vi "Check If Pixels Belong In Sector.vi"() -> (3 "FIFO Timeout?":bool)   [LabVIEW 2013]
uses:
  Globals/Pixel Location Global.vi
  Globals/Accumulated Sector Intensity.vi
  <vilib>/rvi/FIFO/Fifo_Resource/nirvififoEmulationGetNumberOfElementsToWriteFpgaImpl.vi
  <vilib>/rvi/DataTransferAndStorage/Container/Common/niFpgaContainerGetUniqueNameForEmu.vi
  <vilib>/rvi/FIFO/Fifo_Resource/nirvififoEmulationGetNumberOfElementsToReadFpgaImpl.vi
  Globals/Sector Parameter Global.vi
  <vilib>/rvi/FIFO/Fifo_Resource/nirvififoEmulationReadFpgaImpl.vi
  <vilib>/rvi/FIFO/Fifo_Resource/nirvififoEmulationWriteFpgaImpl.vi
  <vilib>/rvi/DataTransferAndStorage/Container/XNode/niFpgaContainer.xnode
  <vilib>/rvi/FIFO/Fifo_Resource/nirvififoEmulationGetNumberOfElementsToWrite.vi
  <vilib>/rvi/FIFO/Fifo_Resource/nirvififoEmulationGetNumberOfElementsToRead.vi
  <vilib>/rvi/FIFO/Fifo_Resource/nirvififoEmulationRead.vi
  <vilib>/rvi/FIFO/Fifo_Resource/nirvififoEmulationWrite.vi
panel:
  out "Number of Elements to Write 4":u32
  out "Number of Elements to Write 3":u32
  out "Number of Elements to Write 2":u32
  out "Number of Elements to Write":u32
  out "Number of Elements to Read 4":u32
  out "Number of Elements to Read 3":u32
  out "Number of Elements to Read 2":u32
  out "Number of Elements to Read":u32
  out "End of  Data?":bool
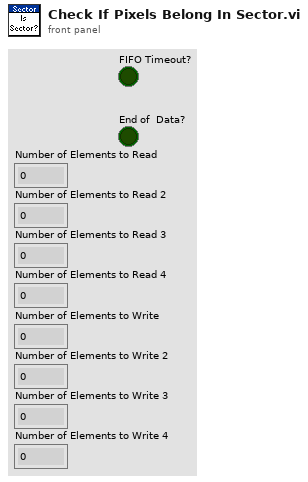
[diagram p1: front panel]
types:
  T1 = cluster{"Pixel Value":u8, "X":fxp<+,11,11>, "Y":fxp<+,11,11>}
  T2 = typedef "Sector Parameter Cluster.ctl" = cluster{"Start Angle":fxp<+/-,17,2>, "End Angle":fxp<+/-,17,2>, "Inner Radius":u16, "Outter Radius":u16, "Hinge X":u16, "Hinge Y":u16, "NumWingSectors":u8}
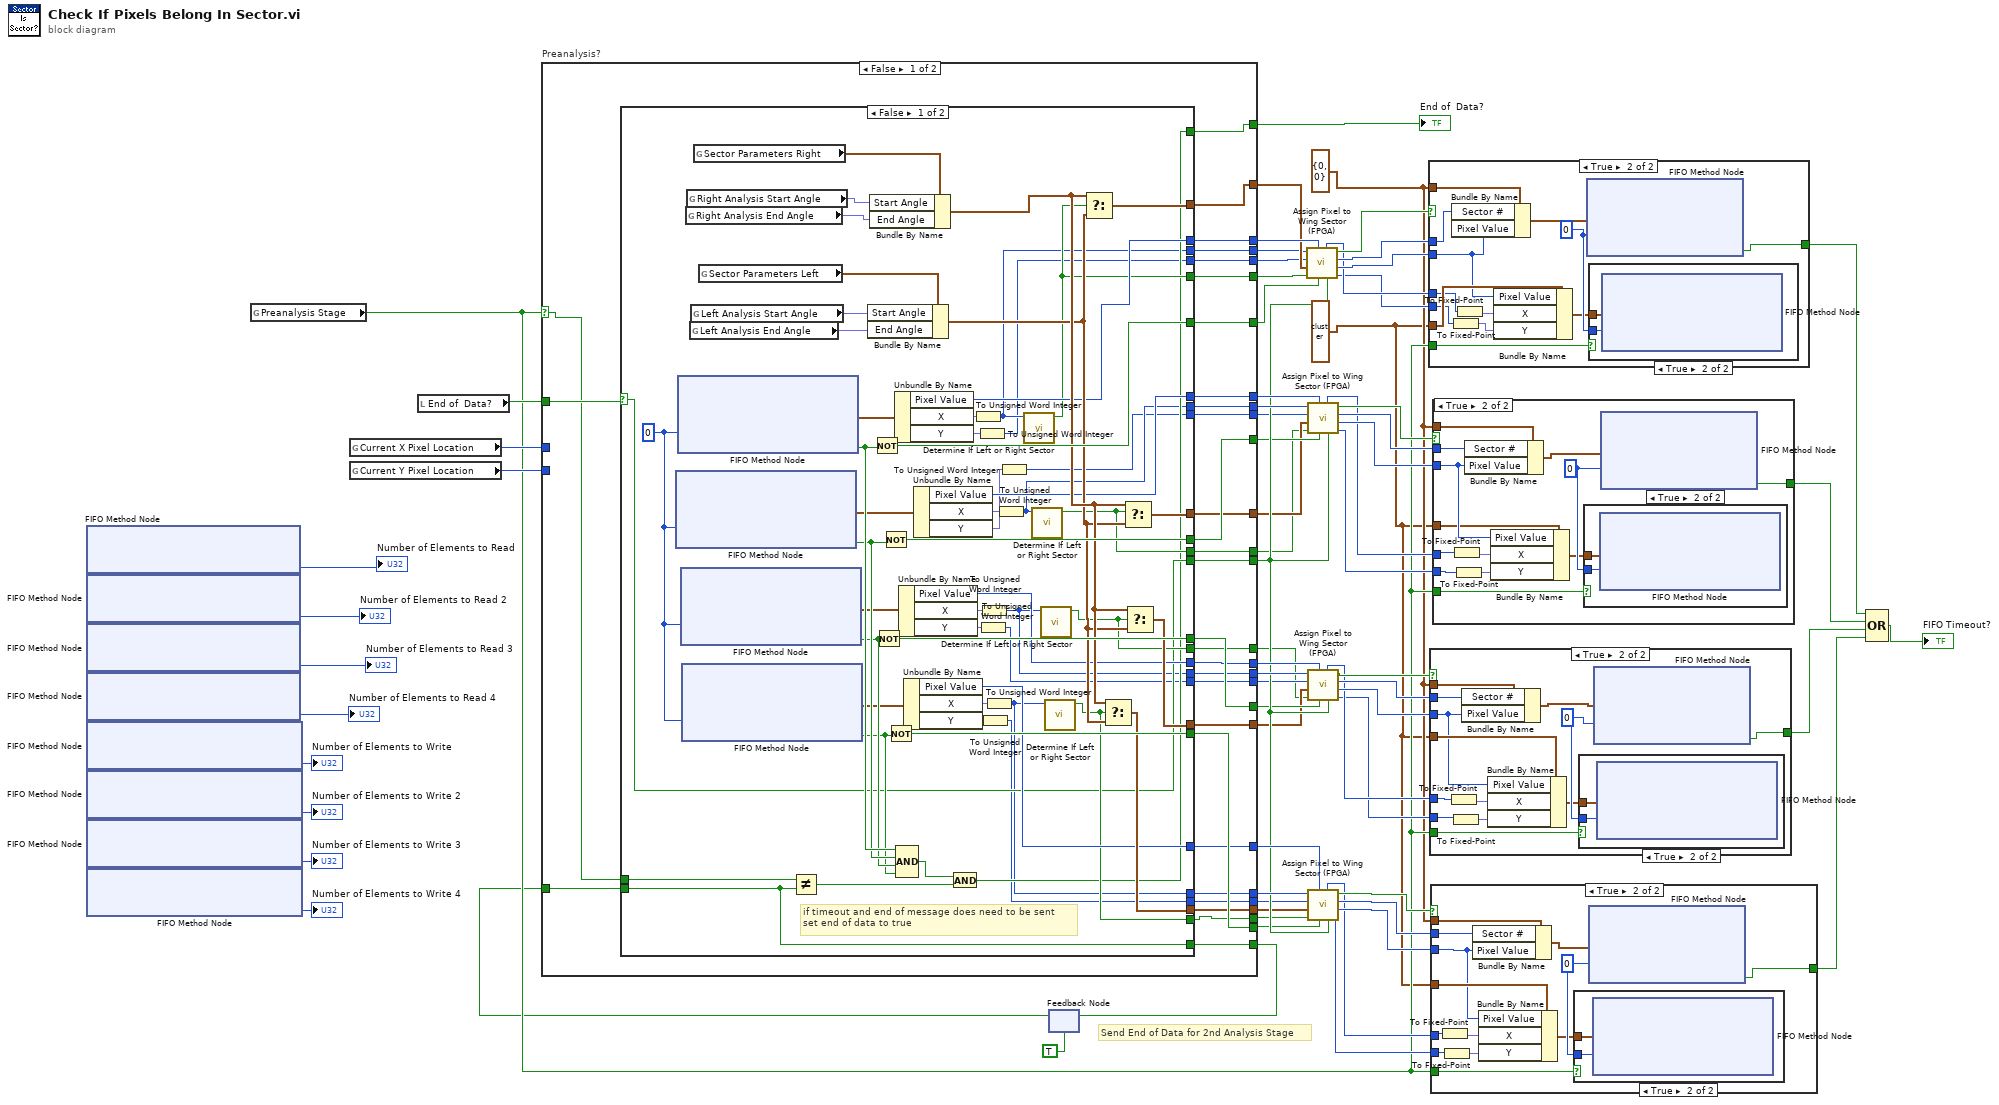
[diagram p0: block diagram]
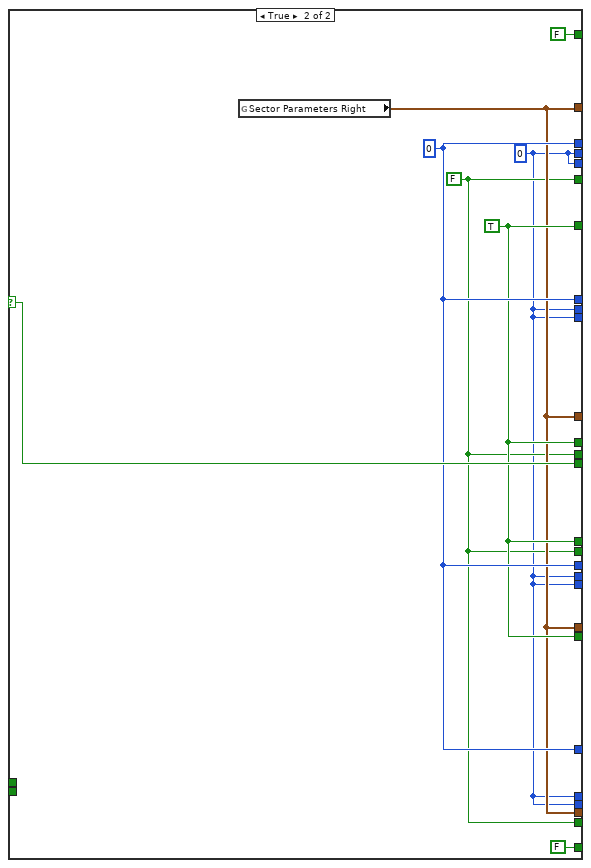
[diagram p2: hidden frame]
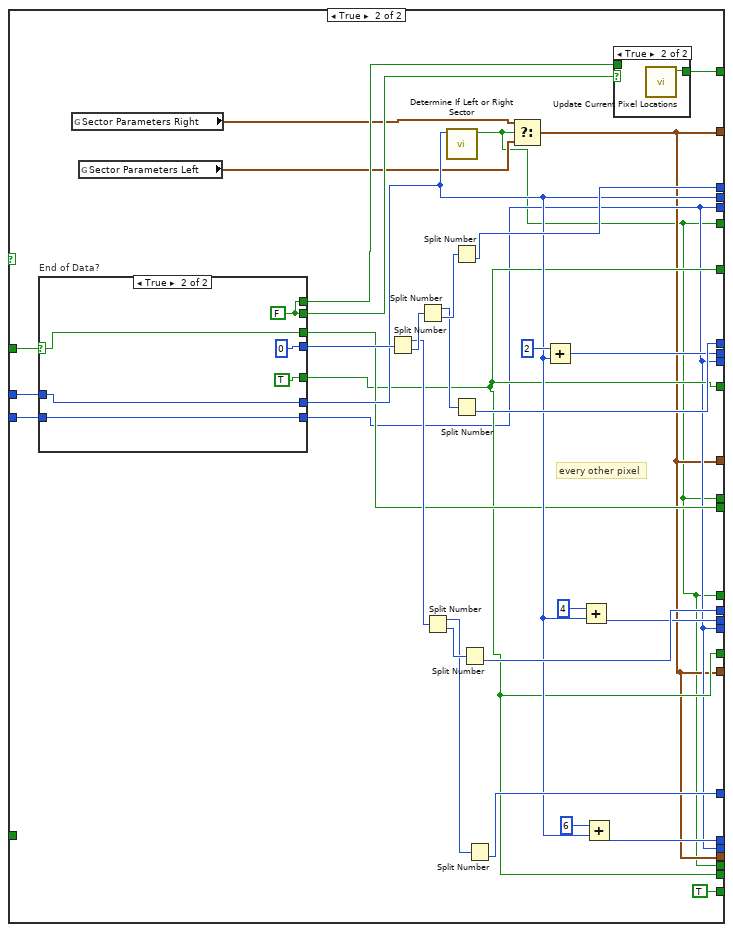
[diagram p3: hidden frame]
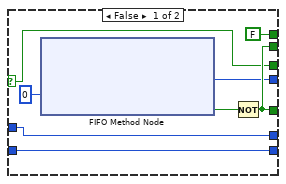
[diagram p4: hidden frame]
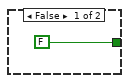
[diagram p6: hidden frame]
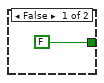
[diagram p8: hidden frame]
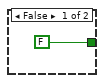
[diagram p10: hidden frame]
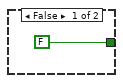
[diagram p12: hidden frame]
diagram:
  w9 = T1 {"Pixel Value"=0, "X"=0.0, "Y"=0.0} ("Element")
  w10 = cluster{"Sector #":u8, "Pixel Value":u8} {"Sector #"=0, "Pixel Value"=0} ("Element")
  # "Send End of Data for 2nd Analysis Stage"
  n1 = xnode ("FIFO Method Node")() -> ("Number of Elements to Read"=→"Number of Elements to Read":u32)  [unwired: 1 in, 1 out]
  n2 = xnode ("FIFO Method Node")() -> ("Number of Elements to Read"=→"Number of Elements to Read 2":u32)  [unwired: 1 in, 1 out]
  n3 = xnode ("FIFO Method Node")() -> ("Number of Elements to Read"=→"Number of Elements to Read 3":u32)  [unwired: 1 in, 1 out]
  n4 = xnode ("FIFO Method Node")() -> ("Number of Elements to Read"=→"Number of Elements to Read 4":u32)  [unwired: 1 in, 1 out]
  n5 = xnode ("FIFO Method Node")() -> ("Number of Elements to Write"=→"Number of Elements to Write":u32)  [unwired: 1 in, 1 out]
  n6 = xnode ("FIFO Method Node")() -> ("Number of Elements to Write"=→"Number of Elements to Write 2":u32)  [unwired: 1 in, 1 out]
  n7 = xnode ("FIFO Method Node")() -> ("Number of Elements to Write"=→"Number of Elements to Write 3":u32)  [unwired: 1 in, 1 out]
  n8 = xnode ("FIFO Method Node")() -> ("Number of Elements to Write"=→"Number of Elements to Write 4":u32)  [unwired: 1 in, 1 out]
  n9 = global read "Accumulated Sector Intensity.vi" "Preanalysis Stage"() -> (w26:bool)
  n10 = global read "Pixel Location Global.vi" "Current X Pixel Location"() -> (w37:u16)
  n11 = global read "Pixel Location Global.vi" "Current Y Pixel Location"() -> (w39:u16)
  n12 = local read "End of  Data?"() -> (w41:bool)
  n13 = feedback #1(TRUE) -> (w12:bool)
  n14 = case "Preanalysis?" shown="False" w26 {
    selector: w26 -> [w70 _]
    tunnel: [w93 w193] -> w68
    tunnel: [w75 w163] -> w50
    tunnel: [w87 w185] -> w49
    tunnel: [w86 w184] -> w48
    tunnel: [w85 w183] -> w47
    tunnel: [w84 w182] -> w46
    tunnel: [w82 w178] -> w45
    tunnel: [w81 w177] -> w44
    tunnel: [w80 w176] -> w43
    tunnel: [w91 w164] -> w42
    tunnel: [w97 w166] -> w27
    tunnel: w41 -> [w98 w173]
    tunnel: [w79 w165] -> w40
    tunnel: w39 -> [_ w172]
    tunnel: [w83 w171] -> w38
    tunnel: w37 -> [_ w170]
    tunnel: [w92 w169] -> w36
    tunnel: [w96 w166] -> w25
    tunnel: [w95 w166] -> w24
    tunnel: [w94 w166] -> w23
    tunnel: [w90 w164] -> w22
    tunnel: [w89 w164] -> w21
    tunnel: [w88 w164] -> w20
    tunnel: [w78 w165] -> w19
    tunnel: [w77 w165] -> w18
    tunnel: [w76 w165] -> w17
    tunnel: [w74 w163] -> w16
    tunnel: [w73 w163] -> w15
    tunnel: [w72 w163] -> w14
    tunnel: w12 -> [w71 _]
    tunnel: [w69 TRUE] -> w11
    frame False {
      n15 = case shown="False" w98 {
        selector: w98 -> [w116 w160]
        tunnel: [w146 w158] -> w97
        tunnel: [w145 w158] -> w96
        tunnel: [w144 w158] -> w95
        tunnel: [w143 w158] -> w94
        tunnel: [w112 FALSE] -> w93
        tunnel: [w116 w160] -> w92
        tunnel: [w138 w157] -> w91
        tunnel: [w137 w157] -> w90
        tunnel: [w136 w157] -> w89
        tunnel: [w133 w157] -> w88
        tunnel: [w132 w159] -> w87
        tunnel: [w131 w159] -> w86
        tunnel: [w130 w159] -> w85
        tunnel: [w129 w159] -> w84
        tunnel: [w110 w155] -> w83
        tunnel: [w108 w155] -> w82
        tunnel: [w106 w155] -> w81
        tunnel: [w104 w155] -> w80
        tunnel: [w109 w155] -> w79
        tunnel: [w107 w155] -> w78
        tunnel: [w105 w155] -> w77
        tunnel: [w103 w155] -> w76
        tunnel: [w120 w156] -> w75
        tunnel: [w119 w156] -> w74
        tunnel: [w118 w156] -> w73
        tunnel: [w117 w156] -> w72
        tunnel: w71 -> [w111 _]
        tunnel: w70 -> [w115 _]
        tunnel: [w111 FALSE] -> w69
        frame False {
          w147 = 0 ("Timeout")
          # "if timeout and end of message does need to be sent\nset end of data to true"
          n16 = xnode ("FIFO Method Node")("Timeout"=w147) -> ("Element"=w102:T1, "Timed Out?"=w141:bool)  [unwired: 1 in, 1 out]
          n17 = xnode ("FIFO Method Node")("Timeout"=w147) -> ("Element"=w101:T1, "Timed Out?"=w142:bool)  [unwired: 1 in, 1 out]
          n18 = xnode ("FIFO Method Node")("Timeout"=w147) -> ("Element"=w100:T1, "Timed Out?"=w140:bool)  [unwired: 1 in, 1 out]
          n19 = xnode ("FIFO Method Node")("Timeout"=w147) -> ("Element"=w99:T1, "Timed Out?"=w139:bool)  [unwired: 1 in, 1 out]
          n20 = global read "Sector Parameter Global.vi" "Right Analysis End Angle"() -> (w151:fxp<+/-,17,2>)
          n21 = global read "Sector Parameter Global.vi" "Right Analysis Start Angle"() -> (w152:fxp<+/-,17,2>)
          n22 = global read "Sector Parameter Global.vi" "Left Analysis End Angle"() -> (w148:fxp<+/-,17,2>)
          n23 = global read "Sector Parameter Global.vi" "Left Analysis Start Angle"() -> (w149:fxp<+/-,17,2>)
          n24 = global read "Sector Parameter Global.vi" "Sector Parameters Right"() -> (w153:T2)
          n25 = global read "Sector Parameter Global.vi" "Sector Parameters Left"() -> (w150:T2)
          n26 = Not Equal?(x=w115, y=w111) -> (x != y?=w113:bool)
          n27 = Bundle By Name(cluster=w150, "Start Angle"=w149, "End Angle"=w148) -> (w134:T2)
          n28 = Bundle By Name(cluster=w153, "Start Angle"=w152, "End Angle"=w151) -> (w135:T2)
          n29 = Not(x=w142) -> (.not. x?=w143:bool)
          n30 = Not(x=w140) -> (.not. x?=w145:bool)
          n31 = Not(x=w141) -> (.not. x?=w144:bool)
          n32 = Not(x=w139) -> (.not. x?=w146:bool)
          n33 = Unbundle By Name(w101) -> ("Pixel Value"=w132:u8, "X"=w128:fxp<+,11,11>, "Y"=w124:fxp<+,11,11>)
          n34 = Compound Arithmetic op=AND(w142, w141, w140, w139) -> (w114:bool)
          n35 = Unbundle By Name(w100) -> ("Pixel Value"=w130:u8, "X"=w126:fxp<+,11,11>, "Y"=w122:fxp<+,11,11>)
          n36 = Unbundle By Name(w99) -> ("Pixel Value"=w129:u8, "X"=w125:fxp<+,11,11>, "Y"=w121:fxp<+,11,11>)
          n37 = Unbundle By Name(w102) -> ("Pixel Value"=w131:u8, "X"=w127:fxp<+,11,11>, "Y"=w123:fxp<+,11,11>)
          n38 = And(x=w114, y=w113) -> (x .and. y?=w112:bool)
          n39 = To Unsigned Word Integer(number=w128) -> (unsigned 16bit integer=w110:u16)
          n40 = To Unsigned Word Integer(number=w124) -> (unsigned 16bit integer=w109:u16)
          n41 = To Unsigned Word Integer(number=w122) -> (unsigned 16bit integer=w105:u16)
          n42 = To Unsigned Word Integer(number=w126) -> (unsigned 16bit integer=w106:u16)
          n43 = To Unsigned Word Integer(number=w121) -> (unsigned 16bit integer=w103:u16)
          n44 = To Unsigned Word Integer(number=w125) -> (unsigned 16bit integer=w104:u16)
          n45 = To Unsigned Word Integer(number=w127) -> (unsigned 16bit integer=w108:u16)
          n46 = To Unsigned Word Integer(number=w123) -> (unsigned 16bit integer=w107:u16)
          n47 = call "Determine If Left or Right Sector.vi"("X Pixel Location"=w110) -> ("Right Sector?"=w120:bool)  [unwired: 10 in]
          n48 = call "Determine If Left or Right Sector.vi"("X Pixel Location"=w108) -> ("Right Sector?"=w119:bool)  [unwired: 10 in]
          n49 = call "Determine If Left or Right Sector.vi"("X Pixel Location"=w106) -> ("Right Sector?"=w118:bool)  [unwired: 10 in]
          n50 = call "Determine If Left or Right Sector.vi"("X Pixel Location"=w104) -> ("Right Sector?"=w117:bool)  [unwired: 10 in]
          n51 = Select(t=w135, s=w120, f=w134) -> (s? t:f=w138:T2)
          n52 = Select(t=w135, s=w117, f=w134) -> (s? t:f=w133:T2)
          n53 = Select(t=w135, s=w119, f=w134) -> (s? t:f=w137:T2)
          n54 = Select(t=w135, s=w118, f=w134) -> (s? t:f=w136:T2)
        }
        frame True {
          w155 = u16 0 ("X")
          w156 = FALSE ("Right Sector?")
          w158 = TRUE
          w159 = u8 0 ("Pixel Value")
          n55 = global read "Sector Parameter Global.vi" "Sector Parameters Right"() -> (w157:T2)
        }
      }
    }
    frame True {
      # "every other pixel"
      n56 = case "End of Data?" shown="True" w173 {
        selector: w173 -> [w195 w202]
        tunnel: [w199 TRUE ("Timed Out?")] -> w166
        tunnel: [w194 u64 0 ("Element")] -> w192
        tunnel: [w199 w205] -> w175
        tunnel: [FALSE ("Timed Out?") w205] -> w174
        tunnel: [w197 w203] -> w165
        tunnel: w172 -> [w197 w203]
        tunnel: [w196 w204] -> w171
        tunnel: w170 -> [w196 w204]
        tunnel: [w195 w202] -> w169
        frame False {
          n57 = xnode ("FIFO Method Node")("Timeout"=0) -> ("Element"=w194:u64, "Timed Out?"=w200:bool)  [unwired: 1 in, 1 out]
          n58 = Not(x=w200) -> (.not. x?=w199:bool)
        }
        frame True {
          w205 = FALSE ("Timed Out?")
        }
      }
      n59 = global read "Sector Parameter Global.vi" "Sector Parameters Right"() -> (w168:T2)
      n60 = global read "Sector Parameter Global.vi" "Sector Parameters Left"() -> (w167:T2)
      n61 = Split Number(x=w192) -> (hi(x)=w190:u32, lo(x)=w191:u32)
      n62 = Split Number(x=w191) -> (hi(x)=w188:u16, lo(x)=w189:u16)
      n63 = Split Number(x=w190) -> (hi(x)=w186:u16, lo(x)=w187:u16)
      n64 = call "Determine If Left or Right Sector.vi"("X Pixel Location"=w171) -> ("Right Sector?"=w163:bool)  [unwired: 10 in]
      n65 = Split Number(x=w189) -> (lo(x)=w185:u8)  [unwired: 1 out]
      n66 = Split Number(x=w188) -> (lo(x)=w184:u8)  [unwired: 1 out]
      n67 = Split Number(x=w187) -> (lo(x)=w183:u8)  [unwired: 1 out]
      n68 = Split Number(x=w186) -> (lo(x)=w182:u8)  [unwired: 1 out]
      n69 = Select(t=w168, s=w163, f=w167) -> (s? t:f=w164:T2)
      n70 = Add(x=u16 2, y=w171) -> (x+y=w178:u16)
      n71 = Add(x=u16 4, y=w171) -> (x+y=w177:u16)
      n72 = Add(x=u16 6, y=w171) -> (x+y=w176:u16)
      n73 = case shown="True" w175 {
        tunnel: [w208 w209] -> w193
        tunnel: w174 -> [w208 _]
        frame False {
        }
        frame True {
          n74 = call "Update Current Pixel Locations.vi"() -> ("End of data?"=w209:bool)  [unwired: 11 in]
        }
      }
    }
  }
  "End of  Data?" <- w68
  n75 = feedback-in #1(w11) -> ()
  n76 = call "Assign Pixel to Wing Sector (FPGA).vi"("End of Data?"=w36, "Valid Data?"=w23, "Pixel Intensity In"=w49, "Right Wing?"=w50, "Sector Parameters"=w42, "Pixel Y"=w40, "Pixel X"=w38) -> ("Y"=w34:u16, "Pixel Intensity Out"=w60:u8, "sector #"=w61:u8, "output valid"=w62:bool, "X"=w35:u16)
  n77 = call "Assign Pixel to Wing Sector (FPGA).vi"("End of Data?"=w36, "Valid Data?"=w24, "Pixel Intensity In"=w48, "Right Wing?"=w16, "Sector Parameters"=w22, "Pixel Y"=w19, "Pixel X"=w45) -> ("Y"=w32:u16, "Pixel Intensity Out"=w57:u8, "sector #"=w58:u8, "output valid"=w59:bool, "X"=w33:u16)
  n78 = call "Assign Pixel to Wing Sector (FPGA).vi"("End of Data?"=w36, "Valid Data?"=w25, "Pixel Intensity In"=w47, "Right Wing?"=w15, "Sector Parameters"=w21, "Pixel Y"=w18, "Pixel X"=w44) -> ("Y"=w30:u16, "Pixel Intensity Out"=w54:u8, "sector #"=w55:u8, "output valid"=w56:bool, "X"=w31:u16)
  n79 = call "Assign Pixel to Wing Sector (FPGA).vi"("End of Data?"=w36, "Valid Data?"=w27, "Pixel Intensity In"=w46, "Right Wing?"=w14, "Sector Parameters"=w20, "Pixel Y"=w17, "Pixel X"=w43) -> ("Y"=w28:u16, "Pixel Intensity Out"=w51:u8, "sector #"=w52:u8, "output valid"=w53:bool, "X"=w29:u16)
  n80 = case shown="True" w62 {
    tunnel: w10 -> [_ w220]
    tunnel: [FALSE ("Timed Out?") w222] -> w66
    tunnel: w61 -> [_ w219]
    tunnel: w60 -> [_ w217]
    tunnel: w35 -> [_ w215]
    tunnel: w34 -> [_ w213]
    tunnel: w26 -> [_ w221]
    tunnel: w9 -> [_ w218]
    frame False {
    }
    frame True {
      w223 = 0 ("Timeout")
      n81 = To Fixed-Point(number=w213) -> (fixed-point=w212:fxp<+,11,11>)  [unwired: 1 in]
      n82 = Bundle By Name(cluster=w220, "Sector #"=w219, "Pixel Value"=w217) -> (w211:cluster{"Sector #":u8, "Pixel Value":u8})
      n83 = To Fixed-Point(number=w215) -> (fixed-point=w214:fxp<+,11,11>)  [unwired: 1 in]
      n84 = Bundle By Name(cluster=w218, "Pixel Value"=w217, "X"=w214, "Y"=w212) -> (w216:T1)
      n85 = xnode ("FIFO Method Node")("Element"=w211, "Timeout"=w223) -> ("Timed Out?"=w222:bool)  [unwired: 1 in, 1 out]
      n86 = case shown="True" w221 {
        tunnel: w223 -> [_ w225]
        tunnel: w216 -> [_ w224]
        frame False {
        }
        frame True {
          n87 = xnode ("FIFO Method Node")("Element"=w224, "Timeout"=w225) -> ()  [unwired: 1 in, 2 out]
        }
      }
    }
  }
  n88 = case shown="True" w56 {
    tunnel: w10 -> [_ w237]
    tunnel: [FALSE ("Timed Out?") w239] -> w64
    tunnel: w55 -> [_ w236]
    tunnel: w54 -> [_ w228]
    tunnel: w31 -> [_ w230]
    tunnel: w30 -> [_ w229]
    tunnel: w26 -> [_ w235]
    tunnel: w9 -> [_ w232]
    frame False {
    }
    frame True {
      w238 = 0 ("Timeout")
      n89 = To Fixed-Point(number=w230) -> (fixed-point=w234:fxp<+,11,11>)  [unwired: 1 in]
      n90 = To Fixed-Point(number=w229) -> (fixed-point=w233:fxp<+,11,11>)  [unwired: 1 in]
      n91 = Bundle By Name(cluster=w237, "Sector #"=w236, "Pixel Value"=w228) -> (w227:cluster{"Sector #":u8, "Pixel Value":u8})
      n92 = Bundle By Name(cluster=w232, "Pixel Value"=w228, "X"=w234, "Y"=w233) -> (w231:T1)
      n93 = case shown="True" w235 {
        tunnel: w238 -> [_ w241]
        tunnel: w231 -> [_ w240]
        frame False {
        }
        frame True {
          n94 = xnode ("FIFO Method Node")("Element"=w240, "Timeout"=w241) -> ()  [unwired: 1 in, 2 out]
        }
      }
      n95 = xnode ("FIFO Method Node")("Element"=w227, "Timeout"=w238) -> ("Timed Out?"=w239:bool)  [unwired: 1 in, 1 out]
    }
  }
  n96 = case shown="True" w53 {
    tunnel: w10 -> [_ w253]
    tunnel: [FALSE ("Timed Out?") w254] -> w63
    tunnel: w52 -> [_ w252]
    tunnel: w51 -> [_ w247]
    tunnel: w29 -> [_ w246]
    tunnel: w28 -> [_ w245]
    tunnel: w26 -> [_ w251]
    tunnel: w9 -> [_ w248]
    frame False {
    }
    frame True {
      w255 = 0 ("Timeout")
      n97 = To Fixed-Point(number=w246) -> (fixed-point=w249:fxp<+,11,11>)  [unwired: 1 in]
      n98 = To Fixed-Point(number=w245) -> (fixed-point=w250:fxp<+,11,11>)  [unwired: 1 in]
      n99 = Bundle By Name(cluster=w253, "Sector #"=w252, "Pixel Value"=w247) -> (w243:cluster{"Sector #":u8, "Pixel Value":u8})
      n100 = Bundle By Name(cluster=w248, "Pixel Value"=w247, "X"=w249, "Y"=w250) -> (w244:T1)
      n101 = case shown="True" w251 {
        tunnel: w255 -> [_ w257]
        tunnel: w244 -> [_ w256]
        frame False {
        }
        frame True {
          n102 = xnode ("FIFO Method Node")("Element"=w256, "Timeout"=w257) -> ()  [unwired: 1 in, 2 out]
        }
      }
      n103 = xnode ("FIFO Method Node")("Element"=w243, "Timeout"=w255) -> ("Timed Out?"=w254:bool)  [unwired: 1 in, 1 out]
    }
  }
  n104 = case shown="True" w59 {
    tunnel: w10 -> [_ w269]
    tunnel: [FALSE ("Timed Out?") w270] -> w65
    tunnel: w58 -> [_ w268]
    tunnel: w57 -> [_ w264]
    tunnel: w33 -> [_ w262]
    tunnel: w32 -> [_ w263]
    tunnel: w26 -> [_ w267]
    tunnel: w9 -> [_ w261]
    frame False {
    }
    frame True {
      w271 = 0 ("Timeout")
      n105 = To Fixed-Point(number=w262) -> (fixed-point=w265:fxp<+,11,11>)  [unwired: 1 in]
      n106 = To Fixed-Point(number=w263) -> (fixed-point=w266:fxp<+,11,11>)  [unwired: 1 in]
      n107 = Bundle By Name(cluster=w269, "Sector #"=w268, "Pixel Value"=w264) -> (w259:cluster{"Sector #":u8, "Pixel Value":u8})
      n108 = Bundle By Name(cluster=w261, "Pixel Value"=w264, "X"=w265, "Y"=w266) -> (w260:T1)
      n109 = case shown="True" w267 {
        tunnel: w271 -> [_ w273]
        tunnel: w260 -> [_ w272]
        frame False {
        }
        frame True {
          n110 = xnode ("FIFO Method Node")("Element"=w272, "Timeout"=w273) -> ()  [unwired: 1 in, 2 out]
        }
      }
      n111 = xnode ("FIFO Method Node")("Element"=w259, "Timeout"=w271) -> ("Timed Out?"=w270:bool)  [unwired: 1 in, 1 out]
    }
  }
  n112 = Compound Arithmetic op=OR(w66, w65, w64, w63) -> (→"FIFO Timeout?":bool)
